vi "aft_Set_Xnode_Configuration.vi"(6 "output type":T1, 8 "error in (no error)":errorcluster, 10 "name/order":string, 11 "diagram in":refnum<vi>) -> (0 "error out":errorcluster, 3 "diagram out":refnum<vi>)   [LabVIEW 2017, in "NI_AdaptiveFilter.lvlib"]
uses:
  <vilib>/addons/Adaptive Filters/NI_AdaptiveFilter.lvlib
  <vilib>/fxp/LVFixedPointRepBitsTypeDef.ctl
  <vilib>/rvi/ClientSDK/Core/Script/FXPMathLib/BaseClass/typeWithOverflowBit.ctl
  <vilib>/rvi/ClientSDK/Core/Script/FXPMathLib/FxpMul/Private/SetOutputType.vi
  <vilib>/rvi/ClientSDK/Core/Script/FXPMathLib/FxpMul/niFpgaHTMathApi_Multiplier.lvclass
  <vilib>/rvi/ClientSDK/Core/Script/FXPMathLib/BaseClass/niFpgaHTMathApi.lvclass
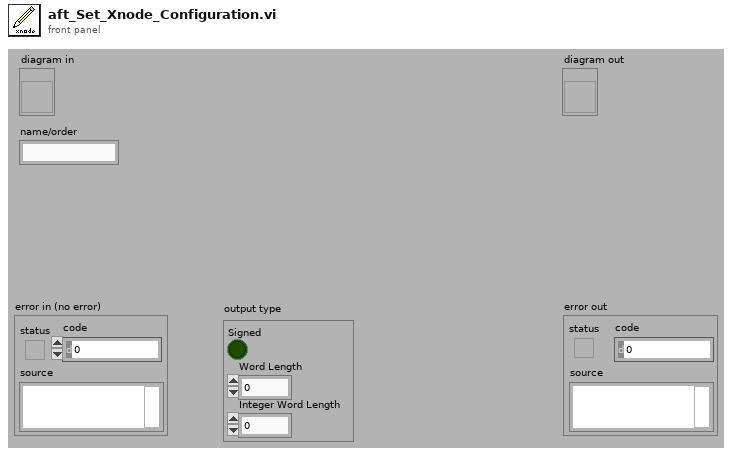
[diagram p1: front panel]
types:
  T1 = typedef "LVFixedPointRepBitsTypeDef.ctl" = cluster{"Signed":bool, "Word Length":u32, "Integer Word Length":i32}
  T2 = typedef "niFpgaHTMathApi.lvclass/typeWithOverflowBit.ctl" = cluster{"type info":T1, "include overflow status?":bool}
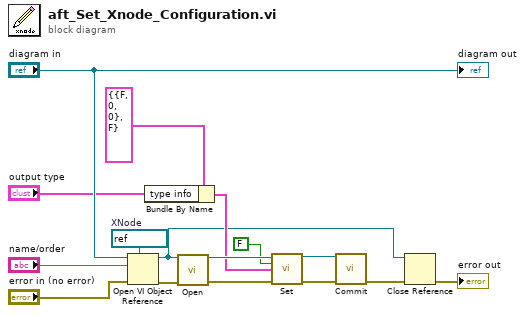
[diagram p0: block diagram]
diagram:
  w15 = refnum<vi> refnum  # XNode
  n1 = Open VI Object Reference(7:w15, 8:"error in (no error)", 10:"name/order", 11:"diagram in") -> (0:w11:errorcluster, 3:w1:refnum<vi>)
  n2 = Bundle By Name(cluster=T2 {"type info"={"Signed"=FALSE, "Word Length"=0, "Integer Word Length"=0}, "include overflow status?"=FALSE} ("x*y type specifics"), "type info"="output type") -> (w5:T2)
  n3 = call <vilib>:"Open.vi"("xnode reference"=w1, "error in (no error)"=w11) -> ("htMultiply out"=w10:refnum<class "niFpgaHTMathApi_Multiplier.lvclass">, "error out"=w9:errorcluster)  [unwired: 12 in]
  n4 = call-poly <vilib>:"Set.vi"("htMultiply in"=w10, "adapt to source"=FALSE, "x*y type specifics"=w5, "error in (no error)"=w9) -> ("htMultiply out"=w4:refnum<class "niFpgaHTMathApi_Multiplier.lvclass">, "error out"=w3:errorcluster)  [unwired: 10 in]
  n5 = call-dynamic "Commit.vi"("htMultiply in"=w4, "error in (no error)"=w3) -> ("error out"=w2:errorcluster)  [unwired: 12 in, 1 out]
  n6 = Close Reference(reference=w1, error in (no error)=w2) -> (error out=→"error out":errorcluster)
  "diagram out" <- "diagram in"
